vi "Potentiometer Control.vi"() -> ()   [LabVIEW 2014]
uses:
  SRE Enum.ctl
panel:
  out "Normalized Value":dbl
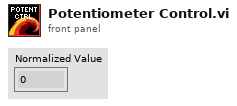
[diagram p1: front panel]
types:
  T1 = typedef "SRE Enum.ctl" = enum16{"Start", "Run", "End"}
  T2 = typedef "WPI_PotentiometerDevRef.ctl" = cluster{"DevStatus":errorcluster, "Controller":T3, "Analog Channel":T4, "Invert Output":bool}
  T3 = typedef "FPGA_TypedefAnalogModule.ctl" = enum16{"Controller 1"}
  T4 = typedef "FPGA_AIChannel.ctl" = enum8{"AI 0", "AI 1", "AI 2", "AI 3", "AI MXP 0", "AI MXP 1", "AI MXP 2", "AI MXP 3", "Invalid"}
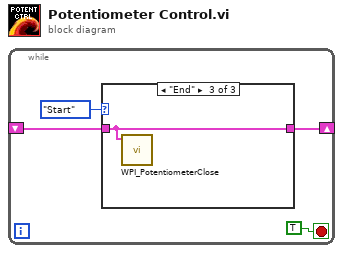
[diagram p0: block diagram]
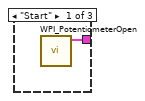
[diagram p2: hidden frame]
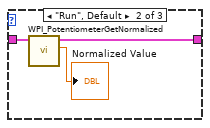
[diagram p3: hidden frame]
diagram:
  n1 = while {
    shift-right: [w3] -> _
    shift-left: _ -> [w2]
    stop <- TRUE stop-if-true
    n2 = case shown="\"End\"" SRE_Enum."Start" ("Enum") {
      tunnel: [w5 w7 w9] -> w3
      tunnel: w2 -> [_ w8 w9]
      frame "Start" {
        n3 = call <vilib>:"WPI_PotentiometerOpen.vi"() -> ("PotDevRef"=w5:T2)  [unwired: 10 in, 1 out]
      }
      frame "Run", Default {
        n4 = call <vilib>:"WPI_PotentiometerGetNormalized.vi"("PotDevRef"=w8) -> ("Normalized Value"=→"Normalized Value":dbl, "PotDevRef"=w7:T2)  [unwired: 8 in, 1 out]
      }
      frame "End" {
        n5 = call <vilib>:"WPI_PotentiometerClose.vi"("PotDevRef"=w9) -> ()  [unwired: 10 in, 1 out]
      }
    }
  }
